vi "Generate Error.vi"(5 "<append> (\"\")":string, 6 "status (T)":bool=TRUE, 7 "<err> (\"\")":string, 8 "error in":errorcluster, 10 "caller name":string, 11 "code":i32) -> (0 "error out":errorcluster)   [LabVIEW 2020, in "Current Value Table(Rebuild).lvlib"]
uses:
  Current Value Table(Rebuild).lvlib
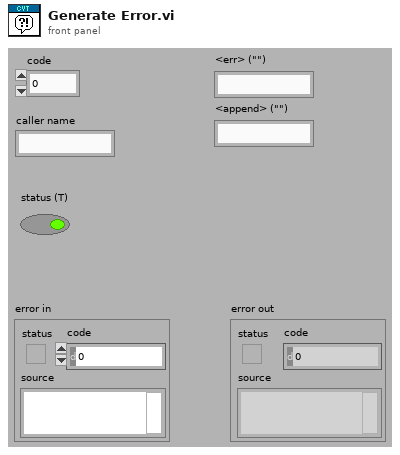
[diagram p1: front panel]
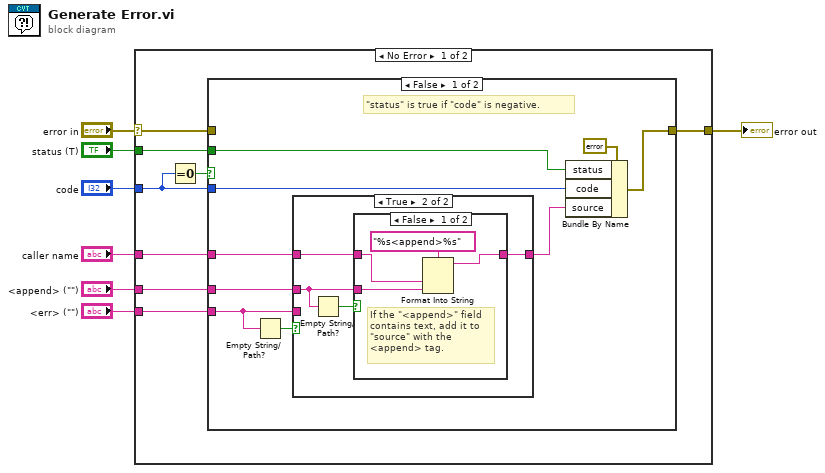
[diagram p0: block diagram]
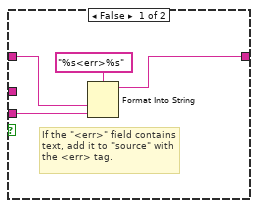
[diagram p2: hidden frame]
diagram:
  n1 = case shown="No Error" "error in" {
    selector: "error in" -> [w13 w39]
    tunnel: [w14 w39] -> w2
    tunnel: "code" -> [w12 _]
    tunnel: "caller name" -> [w15 _]
    tunnel: "<err> (\"\")" -> [w11 _]
    tunnel: "<append> (\"\")" -> [w10 _]
    tunnel: "status (T)" -> [w8 _]
    frame No Error {
      n2 = Equal To 0?(x=w12) -> (x = 0?=w9:bool)
      n3 = case shown="False" w9 {
        tunnel: w13 -> [_ w38]
        tunnel: w15 -> [w16 _]
        tunnel: [w24 w38] -> w14
        tunnel: w12 -> [w23 _]
        tunnel: w11 -> [w21 _]
        tunnel: w10 -> [w20 _]
        tunnel: w8 -> [w17 _]
        frame False {
          # "\"status\" is true if \"code\" is negative."
          n4 = Empty String/Path?(string/path=w21) -> (empty?=w22:bool)
          n5 = case shown="True" w22 {
            tunnel: w16 -> [w25 w30]
            tunnel: w21 -> [w26 _]
            tunnel: w20 -> [_ w31]
            tunnel: [w27 w29] -> w19
            frame False {
              # "If the \"<err>\" field contains text, add it to \"source\" with the <err> tag."
              n6 = Format Into String(format string="%s<err>%s", w25, w26) -> (resulting string=w27:string)  [unwired: 2 in, 1 out]
            }
            frame True {
              n7 = Empty String/Path?(string/path=w31) -> (empty?=w32:bool)
              n8 = case shown="False" w32 {
                tunnel: w31 -> [w35 _]
                tunnel: w30 -> [w36 w37]
                tunnel: [w33 w37] -> w29
                frame False {
                  # "If the \"<append>\" field contains text, add it to \"source\" with the <append> tag."
                  n9 = Format Into String(format string="%s<append>%s", w36, w35) -> (resulting string=w33:string)  [unwired: 2 in, 1 out]
                }
                frame True {
                }
              }
            }
          }
          n10 = Bundle By Name(cluster=errorcluster {"status"=FALSE, "code"=0, "source"=""} ("error IO"), "status"=w17, "code"=w23, "source"=w19) -> (w24:errorcluster)
        }
        frame True {
          # "Do nothing if the new code is zero."
        }
      }
    }
    frame Error {
      # "Do nothing if there is already an error on the wire."
    }
  }
  "error out" <- w2
